vi "Configure OVP.vi"(0 "VISA resource name":refnum<visa-resource-name>, 2 "Enable OVP (T: Enable)":bool=TRUE, 5 "Address (0)":dbl min=0.0 max=31.0 step=1.0 format="%#.0p", 7 "Voltage Limit (80.000 V)":dbl=80.0 min=0.0 max=150.0 step=0.001 format="%.3g", 9 "Protection Delay (0.001)":dbl=0.001 min=0.001 max=0.6 step=0.001 format="%.3g", 11 "error in (no error)":errorcluster) -> (4 "VISA resource name out":refnum<visa-resource-name>, 15 "error out":errorcluster)   [LabVIEW 2020, in "BK Precision 911X Series.lvlib"]
doc: "Configures over voltage protection (OVP) of the power supply."
uses:
  BK Precision 911X Series.lvlib
panel:
  # "s"
  # "V"
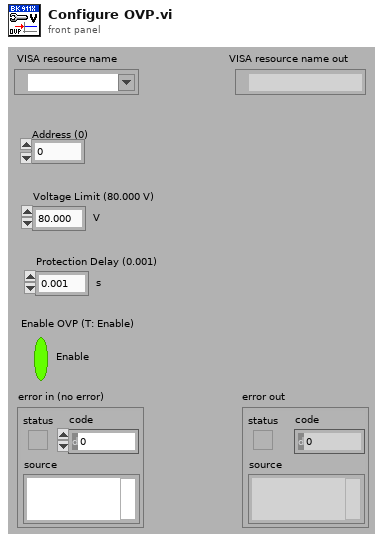
[diagram p1: front panel]
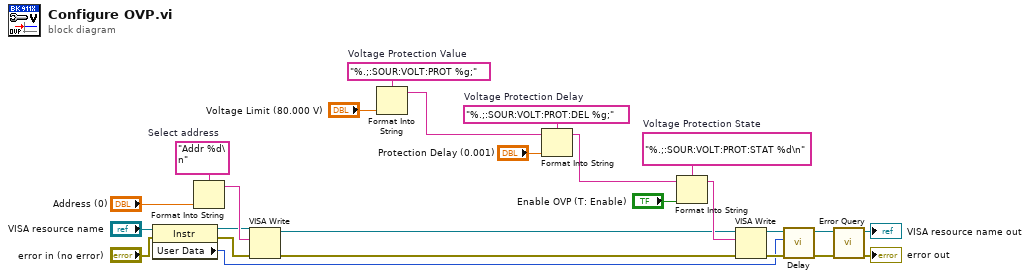
[diagram p0: block diagram]
diagram:
  w16 = "%.;:SOUR:VOLT:PROT:DEL %g;"  # Voltage Protection Delay
  w20 = "%.;:SOUR:VOLT:PROT:STAT %d\n"  # Voltage Protection State
  w22 = "Addr %d\n"  # Select address
  w21 = "%.;:SOUR:VOLT:PROT %g;"  # Voltage Protection Value
  n1 = property class="Instr"(reference="VISA resource name", error in="error in (no error)") -> (reference out=w3:refnum<visa-resource-name>, error out=w2:errorcluster, "User Data"=w1:u32)
  n2 = Format Into String(format string=w22, "Address (0)") -> (resulting string=w23:string)  [unwired: 2 in, 1 out]
  n3 = VISA Write(VISA resource name=w3, write buffer=w23, error in (no error)=w2) -> (VISA resource name out=w11:refnum<visa-resource-name>, error out=w10:errorcluster)  [unwired: 1 out]
  n4 = Format Into String(format string=w21, "Voltage Limit (80.000 V)") -> (resulting string=w13:string)  [unwired: 2 in, 1 out]
  n5 = Format Into String(format string=w16, initial string=w13, "Protection Delay (0.001)") -> (resulting string=w12:string)  [unwired: 1 in, 1 out]
  n6 = Format Into String(format string=w20, initial string=w12, "Enable OVP (T: Enable)") -> (resulting string=w19:string)  [unwired: 1 in, 1 out]
  n7 = VISA Write(VISA resource name=w11, write buffer=w19, error in (no error)=w10) -> (VISA resource name out=w9:refnum<visa-resource-name>, error out=w8:errorcluster)  [unwired: 1 out]
  n8 = call "Delay.vi"("error in (no error)"=w8, "Delay Time (0 ms)"=w1, "VISA resource name"=w9) -> ("error out"=w7:errorcluster, "VISA resource name out"=w6:refnum<visa-resource-name>)  [unwired: 7 in]
  n9 = call "Error Query.vi"("error in (no error)"=w7, "VISA resource name"=w6) -> ("error out"=→"error out":errorcluster, "VISA resource name out"=→"VISA resource name out":refnum<visa-resource-name>)  [unwired: 6 in, 2 out]
